vi "NIIE_Circle.vi"(6 "Fill Color":u32(colorbox), 7 "Fill?(F)":bool, 8 "Error":errorcluster, 9 "Edge Color":u32(colorbox), 11 "Rect":T1) -> (0 "Error Out":errorcluster, 3 "New Picture Out":picture)   [LabVIEW 2021]
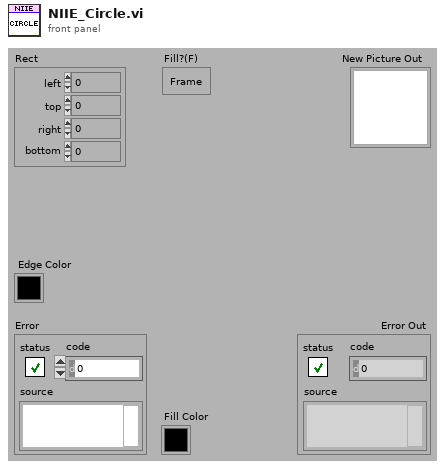
[diagram p1: front panel]
types:
  T1 = cluster{"left":i16, "top":i16, "right":i16, "bottom":i16}
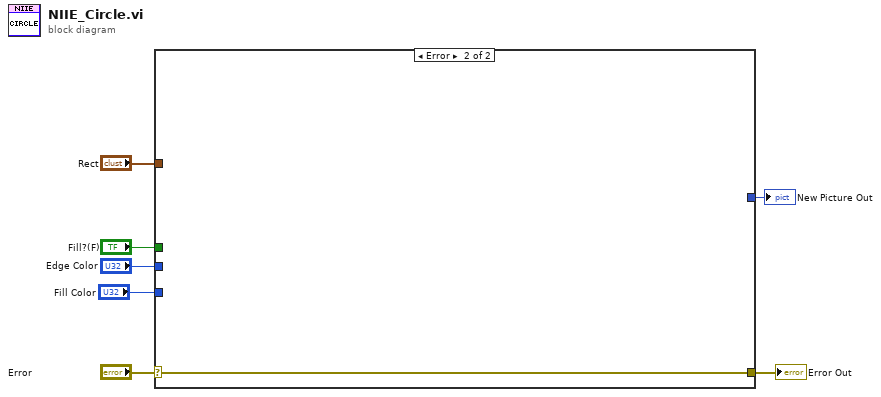
[diagram p0: block diagram]
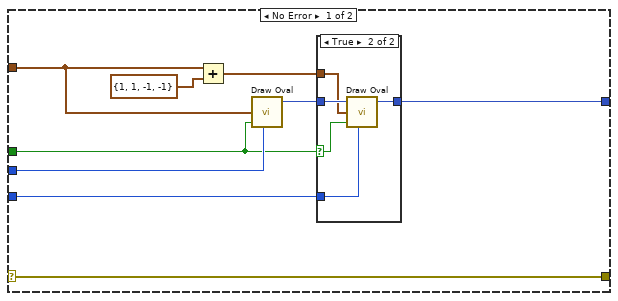
[diagram p2: hidden frame]
diagram:
  n1 = case shown="Error" "Error" {
    selector: "Error" -> [w16 w23]
    tunnel: [w16 w23] -> w6
    tunnel: [w12 _] -> w5
    tunnel: "Rect" -> [w10 _]
    tunnel: "Fill?(F)" -> [w14 _]
    tunnel: "Edge Color" -> [w15 _]
    tunnel: "Fill Color" -> [w11 _]
    frame No Error {
      n2 = Add(x=w10, y=T1 {"left"=1, "top"=1, "right"=-1, "bottom"=-1}) -> (x+y=w8:T1)
      n3 = call <vilib>:"Draw Oval.vi"("rect"=w10, "fill?(F)"=w14, "color(black)"=w15) -> ("new picture"=w13:picture)  [unwired: 2 in, 4 out]
      n4 = case shown="True" w14 {
        selector: w14 -> [_ w18]
        tunnel: w13 -> [w17 w22]
        tunnel: [w17 w21] -> w12
        tunnel: w11 -> [_ w20]
        tunnel: w8 -> [_ w19]
        frame False {
        }
        frame True {
          n5 = call <vilib>:"Draw Oval.vi"("picture"=w22, "rect"=w19, "fill?(F)"=w18, "color(black)"=w20) -> ("new picture"=w21:picture)  [unwired: 1 in, 4 out]
        }
      }
    }
    frame Error {
    }
  }
  "Error Out" <- w6
  "New Picture Out" <- w5
